vi "writeToXML.vi"(8 "error in (no error)":errorcluster, 10 "ClassLabel":string, 11 "WSMode in":refnum<class "WSMode.lvclass">) -> (0 "error out":errorcluster, 2 "XMLout":string, 3 "WSMode out":refnum<class "WSMode.lvclass">)   [LabVIEW 2022 SP3, in "TCSDataDefinitions.lvlib" / "TCSWeatherServerCommand.lvlib" / "WSMode.lvclass"]
uses:
  WSMode.lvclass
  WSMode.lvclass/WSMode.ctl
  TCSWeatherServerCommand/TCSWeatherServerCommand.lvclass
  <userlib>/Common/XML/XMLGenerator/XMLGenerator.lvclass
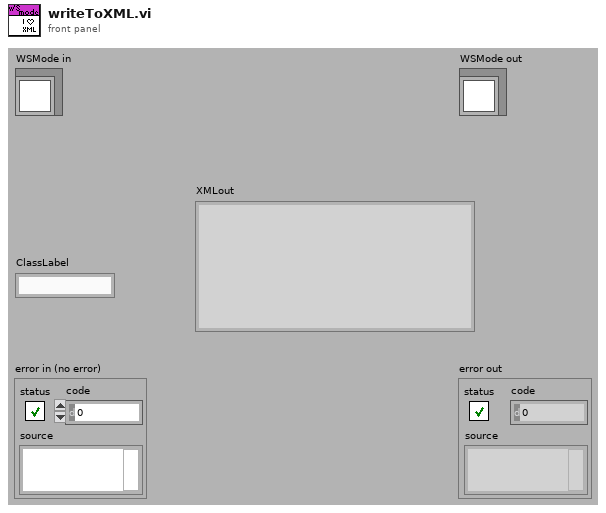
[diagram p1: front panel]
types:
  T1 = typedef "TCSDataDefinitions.lvlib/TCSWeatherServerCommand.lvlib/wsMode.ctl" = enum16{"Automatic", "Manual"}
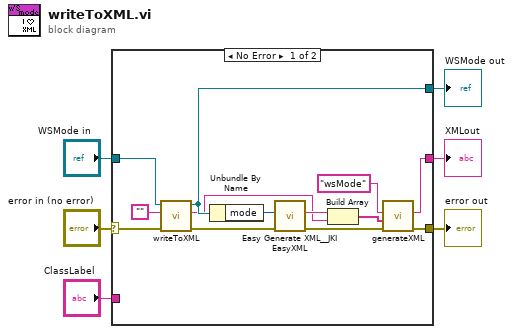
[diagram p0: block diagram]
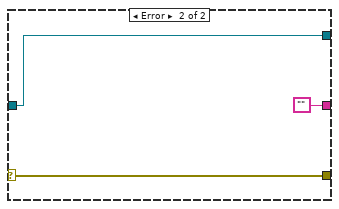
[diagram p2: hidden frame]
diagram:
  n1 = case shown="No Error" "error in (no error)" {
    selector: "error in (no error)" -> [w11 w22]
    tunnel: [w10 w22] -> w5
    tunnel: [w17 w21] -> w3
    tunnel: "WSMode in" -> [w18 w21]
    tunnel: [w9 ""] -> w2
    tunnel: "ClassLabel" -> [_ _]
    frame No Error {
      n2 = call-parent "writeToXML.vi"("error in (no error)"=w11, "ClassLabel"="", "TCSWeatherServerCommand in"=w18) -> ("error out"=w13:errorcluster, "XMLout"=w14:string, "TCSWeatherServerCommand out"=w17:refnum<class "WSMode.lvclass">)  [unwired: 6 in]
      n3 = Unbundle By Name(w17) -> ("mode"=w16:T1)
      n4 = call <vilib>:"Easy Generate XML__JKI EasyXML.vi"("error in (no error)"=w13, "LabVIEW Data"=w16) -> ("error out"=w12:errorcluster, "XML String"=w15:string)  [unwired: 8 in]
      n5 = Build Array(w15, w14) -> (w7:string[])
      n6 = call <userlib>:"generateXML.vi"("error in"=w12, "childrenXML"=w7, "elementName"="wsMode" ("Class Label")) -> ("error out"=w10:errorcluster, "XML out"=w9:string)  [unwired: 6 in, 1 out]
    }
    frame Error {
    }
  }
  "error out" <- w5
  "WSMode out" <- w3
  "XMLout" <- w2
